vi "Data Readers and Writers.vi"(5 "Calling VI Ref":refnum<vi>, 8 "error in (no error)":errorcluster, 9 "Full Element Name":string[](array[string]), 11 "JKI SM in":refnum<class "JKI SM.lvclass">) -> (0 "error out":errorcluster)   [LabVIEW 2020]
uses:
  <userlib>/_OpenG.lib/comparison/comparison.llb/openg_comparison__ogtk.lvlib
  JKI State Machine API/source/JKI SM/JKI SM.lvclass
  <vilib>/regexp/Match Regular Expression.xnode
  <userlib>/_OpenG.lib/comparison/comparison.llb/I32 Changed__ogtk.vi
  <userlib>/_OpenG.lib/comparison/comparison.llb/Boolean Changed__ogtk.vi
  <userlib>/_OpenG.lib/error/error.llb/openg_error.lvlib
  <userlib>/_OpenG.lib/error/error.llb/Filter Error Codes (Array)__ogtk.vi
  <userlib>/_OpenG.lib/string/string.llb/openg_string.lvlib
panel:
  in  "Listbox":i32(listbox)
  in  "OK":bool
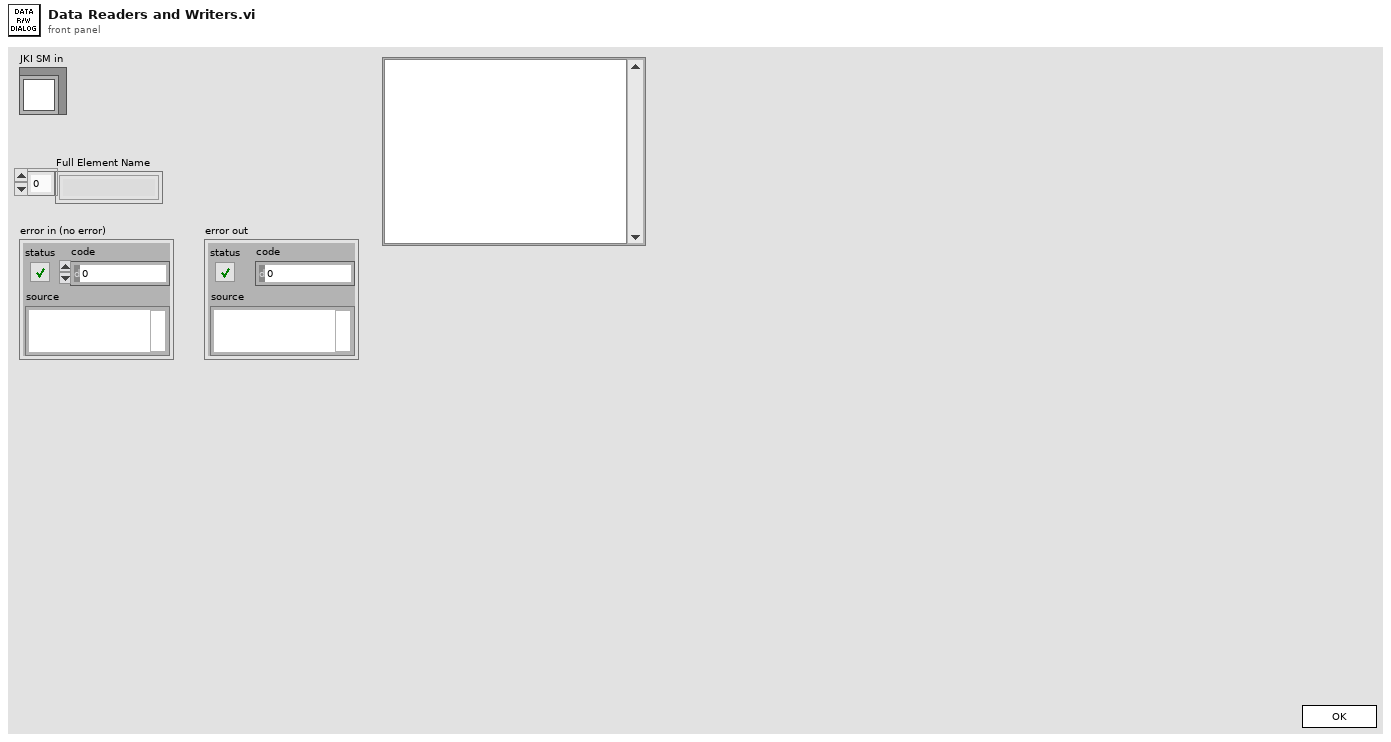
[diagram p1: front panel]
types:
  T1 = enum32{"Invalid", "Standard", "Closed", "Hidden", "Minimized", "Maximized"}
  T2 = enum32{"invalid app kind", "Development System", "Run Time System", "Student Edition", "Embedded LabVIEW", "Evaluation", "Custom"}
  T3 = enum32{"Invalid", "Default", "Floating", "Floating/Auto-Hide", "Modal"}
  T4 = cluster{"Core":cluster{"Current VI Reference":refnum<vi>, "Close Panel on Exit?":bool}, "Your Boolean data":bool, "Your string data":string, "JKI SM in":refnum<class "JKI SM.lvclass">, "Full Element Name":string[]}
  T5 = typedef "LVPoint32TypeDef.ctl" = cluster{"Horizontal":i32, "Vertical":i32}
  T6 = cluster{"Shift":bool, "Ctrl":bool, "Alt":bool, "Cmd":bool, "Opt":bool}
  T7 = cluster{"StringConstant":refnum<vi>, "Structure":string, "Frame Name":string, "State Call":string}[]
  T8 = cluster{"Current VI Reference":refnum<vi>, "Close Panel on Exit?":bool}
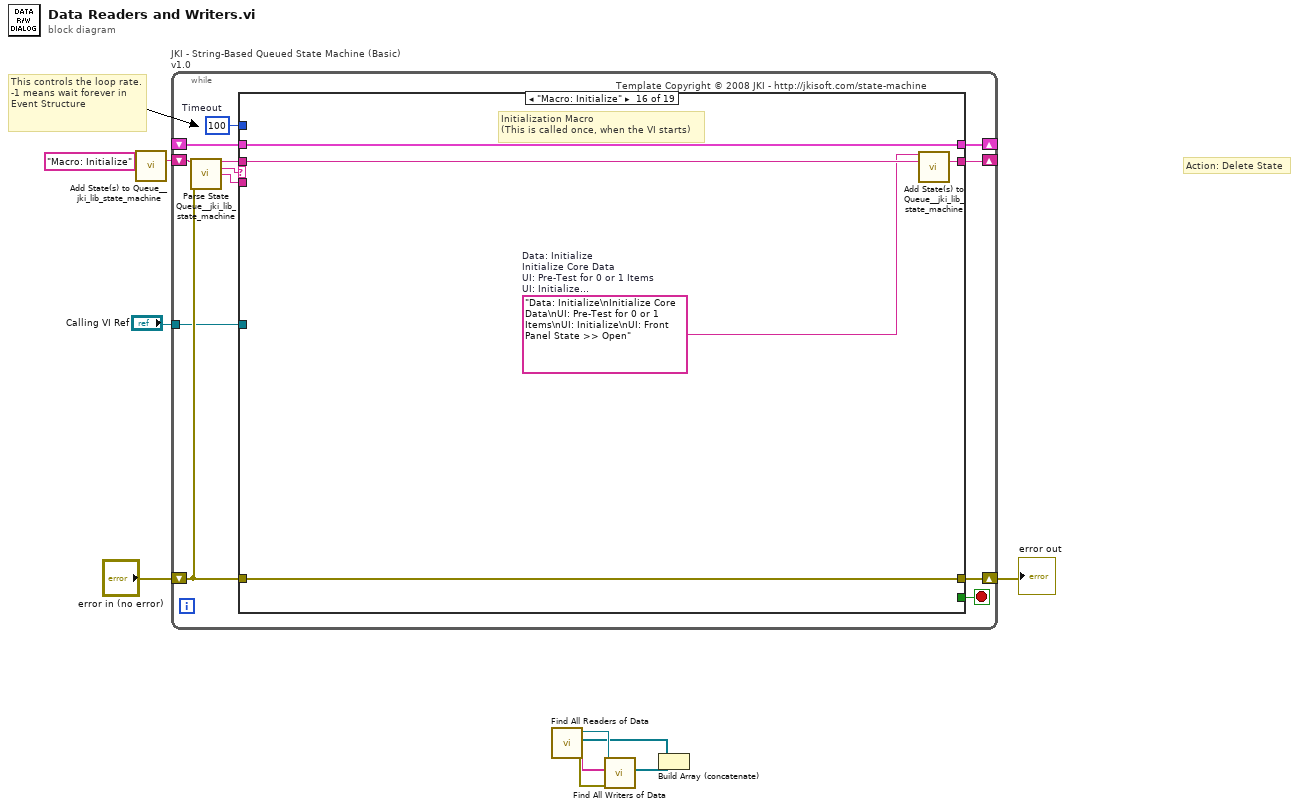
[diagram p0: block diagram]
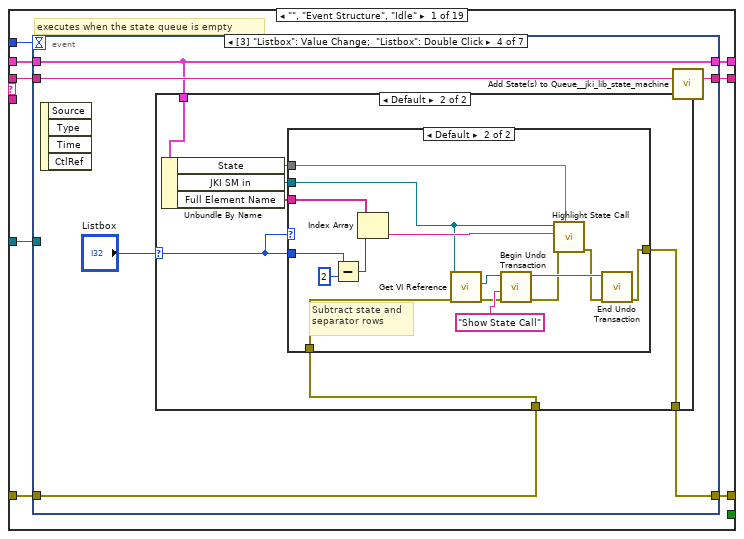
[diagram p2: hidden frame]
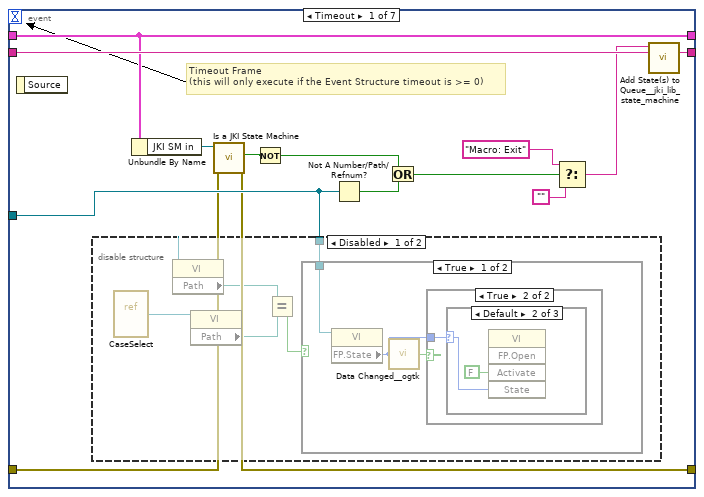
[diagram p3: hidden frame]
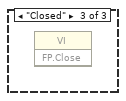
[diagram p6: hidden frame]
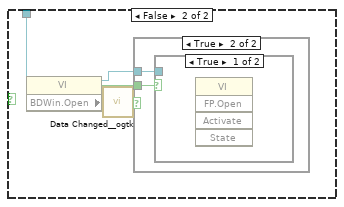
[diagram p7: hidden frame]
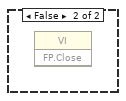
[diagram p9: hidden frame]
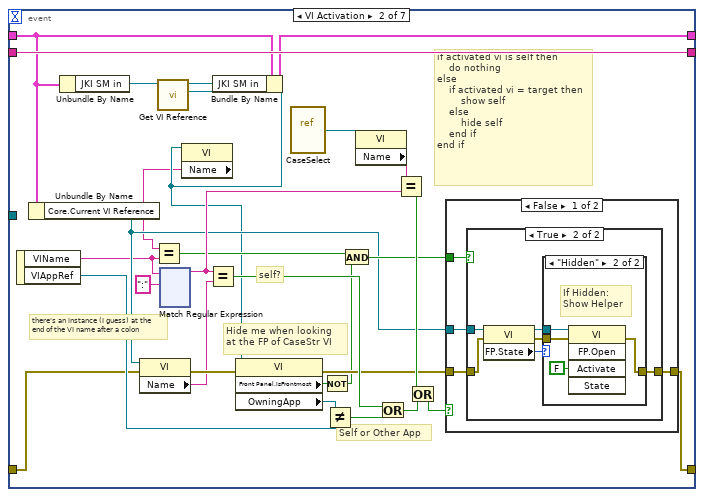
[diagram p11: hidden frame]
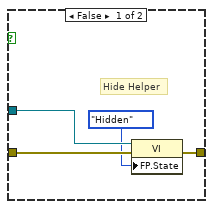
[diagram p12: hidden frame]
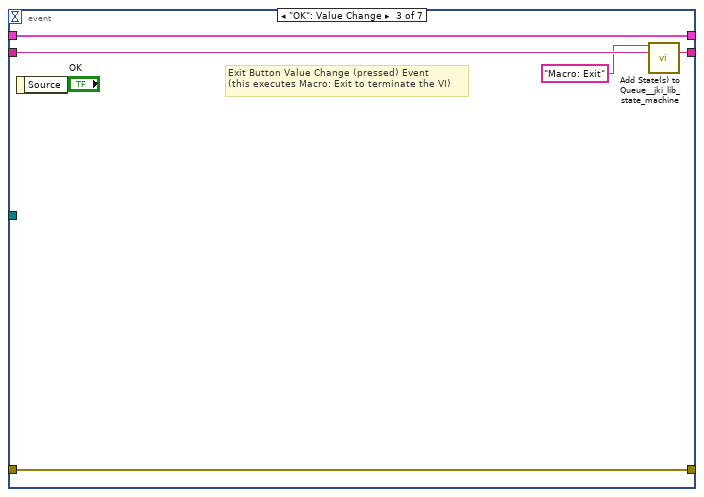
[diagram p15: hidden frame]
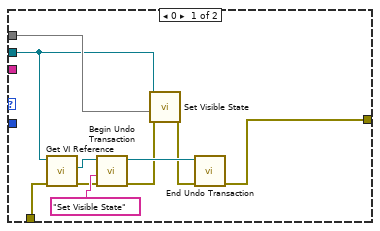
[diagram p17: hidden frame]
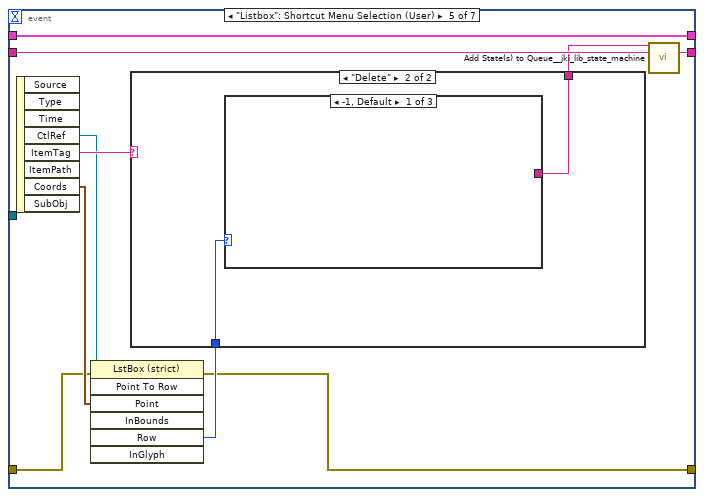
[diagram p18: hidden frame]
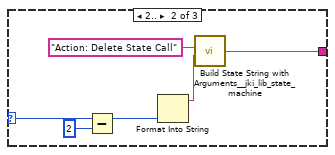
[diagram p20: hidden frame]
diagram:
  # "Action: Delete State"
  # "This controls the loop rate. -1 means wait forever in Event Structure"
  n1 = call <vilib>:"Add State(s) to Queue__jki_lib_state_machine.vi"("State(s) in (\"\")"="Macro: Initialize") -> ("States Out"=w12:string)  [unwired: 14 in]
  n2 = while "JKI - String-Based Queued State Machine (Basic) v1.0" {
    shift-right: [w17] -> _
    shift-left: _ -> [w16]
    shift-right: [w20] -> w10
    shift-left: "error in (no error)" -> [w14]
    shift-right: [w19] -> _
    shift-left: w12 -> [w21]
    tunnel: "Calling VI Ref" -> [w13]
    stop <- w18 stop-if-true
    w15 = 100  # Timeout
    # "Template Copyright © 2008 JKI - http://jkisoft.com/state-machine"
    n3 = call <vilib>:"Parse State Queue__jki_lib_state_machine.vi"("State Queue"=w21, "Error In (no error)"=w14) -> ("Remaining States"=w23:string, "Current State"=w24:string, "Arguments"=w22:string)  [unwired: 11 in]
    n4 = case shown="\"Macro: Initialize\"" w24 {
      selector: w24 -> [_ _ w376 _ _ _ _ _ _ _ _ _ _ _ _ _ _ _ _]
      tunnel: w23 -> [w32 w375 w380 w400 w411 w416 w420 w429 w436 w440 w459 w476 w495 w506 w535 w540 w550 w554 w558]
      tunnel: w22 -> [_ _ _ _ _ _ _ _ _ _ _ _ w490 w500 _ _ _ _ _]
      tunnel: w16 -> [w30 w372 w378 w392 w408 w414 w417 _ w433 w437 w456 w470 w493 w502 w532 w538 w547 w551 w555]
      tunnel: [w29 w373 w382 w387 errorcluster {"status"=FALSE, "code"=0, "source"=""} ("error out") w413 w418 w426 w431 w438 w457 w467 w491 w503 w533 w536 w548 w552 w556] -> w20
      tunnel: w14 -> [w28 w373 w381 w388 w406 w413 w418 w426 w430 w438 w457 w468 w492 w504 w533 w536 w548 w552 w556]
      tunnel: [w31 w374 w379 w399 w410 w415 w419 w428 w435 w439 w458 w475 w494 w505 w534 w539 w549 w553 w557] -> w19
      tunnel: [_ _ _ _ _ TRUE _ _ _ _ _ _ _ _ _ _ _ _ _] -> w18
      tunnel: [w27 w372 w378 w398 w408 w414 w417 w427 w433 w437 w456 w470 w493 w502 w532 w538 w547 w551 w555] -> w17
      tunnel: w15 -> [w26 _ _ _ _ _ _ _ _ _ _ _ _ _ _ _ _ _ _]
      tunnel: w13 -> [w25 _ _ _ _ _ _ _ _ _ _ _ _ _ _ _ _ _ _]
      frame "", "Event Structure", "Idle" {
        # "executes when the state queue is empty"
        n5 = event shown="[3] \"Listbox\": Value Change;  \"Listbox\": Double Click" {
          selector: _ -> [_ _ _ _ _ _ _]
          dyn-events: _ -> [_ _ _ _ _ _ _]
          timeout: w26 -> [_ _ _ _ _ _ _]
          tunnel: w32 -> [w46 w92 w228 w234 w277 w297 w371]
          tunnel: [w45 w92 w227 w233 w276 w296 w370] -> w31
          tunnel: w30 -> [w40 w66 w225 w232 w269 w295 w368]
          tunnel: [w35 w67 w226 w230 w268 w290 w369] -> w29
          tunnel: w28 -> [w36 w68 w226 w231 w271 w291 w369]
          tunnel: [w40 w65 w225 w232 w269 w295 w368] -> w27
          tunnel: w25 -> [w41 _ _ _ _ _ _]
          event Timeout {
            # "Timeout Frame\n(this will only execute if the Event Structure timeout is >= 0)"
            n6 = event-data() -> ()  [unwired: 1 in, 1 out]
            n7 = disable-structure shown="Disabled" {
              disable-tunnel: w41 -> [w47 _]
              frame Disabled {
                n8 = vi-ref "CaseSelect.vi"() -> (w49:refnum<vi>)
                n9 = property class="VI"(reference=w47) -> ("Path"=w48:path)  [unwired: 1 in, 2 out]
                n10 = property class="VI"(reference=w49) -> ("Path"=w51:path)  [unwired: 1 in, 2 out]
                n11 = Equal?(x=w48, y=w51) -> (x = y?=w50:bool)
                n12 = case shown="True" w50 {
                  tunnel: w47 -> [w52 w59]
                  frame True {
                    n13 = property class="VI"(reference=w52) -> ("FP.State"=w53:T1)  [unwired: 1 in, 2 out]
                    n14 = call-poly <userlib>:"Data Changed__ogtk.vi"("I32"=w53) -> ("Changed"=w54:bool)
                    n15 = case shown="True" w54 {
                      tunnel: w53 -> [_ w55]
                      frame False {
                      }
                      frame True {
                        n16 = case shown="Default" w55 {
                          selector: w55 -> [_ w56 _]
                          frame "Invalid" {
                          }
                          frame Default {
                            n17 = invoke class="VI" method="FP.Open"("Activate"=FALSE ("Activate?"), "State"=w56) -> ()  [unwired: 3 in, 5 out]
                          }
                          frame "Closed" {
                            n18 = invoke class="VI" method="FP.Close"() -> ()  [unwired: 3 in, 3 out]
                          }
                        }
                      }
                    }
                  }
                  frame False {
                    n19 = property class="VI"(reference=w59) -> (reference out=w58:refnum<vi>, "BDWin.Open"=w60:bool)  [unwired: 1 in, 1 out]
                    n20 = call-poly <userlib>:"Data Changed__ogtk.vi"("Boolean"=w60) -> ("Changed"=w61:bool)
                    n21 = case shown="True" w61 {
                      tunnel: w60 -> [_ w63]
                      tunnel: w58 -> [_ w62]
                      frame False {
                      }
                      frame True {
                        n22 = case shown="True" w63 {
                          tunnel: w62 -> [_ _]
                          frame True {
                            n23 = invoke class="VI" method="FP.Open"() -> ()  [unwired: 5 in, 5 out]
                          }
                          frame False {
                            n24 = invoke class="VI" method="FP.Close"() -> ()  [unwired: 3 in, 3 out]
                          }
                        }
                      }
                    }
                  }
                }
              }
              frame Enabled {
              }
            }
            n25 = Unbundle By Name(w40) -> ("JKI SM in"=w39:refnum<class "JKI SM.lvclass">)
            n26 = call "Is a JKI State Machine.vi"("error in (no error)"=w36, "JKI SM in"=w39) -> ("error out"=w35:errorcluster, "Is a JKI State Machine"=w38:bool)  [unwired: 7 in, 1 out]
            n27 = Not(x=w38) -> (.not. x?=w37:bool)
            n28 = Not A Number/Path/Refnum?(number/path/refnum=w41) -> (NaN/Path/Refnum?=w34:bool)
            n29 = Or(x=w37, y=w34) -> (x .or. y?=w33:bool)
            n30 = Select(t="Macro: Exit", s=w33, f="") -> (s? t:f=w42:string)
            n31 = call <vilib>:"Add State(s) to Queue__jki_lib_state_machine.vi"("State(s) in Front (\"\")"=w42, "State(s) in (\"\")"=w46) -> ("States Out"=w45:string)  [unwired: 13 in]
          }
          event VI Activation {
            # "Self or Other App"
            # "self?"
            # "Hide me when looking\nat the FP of CaseStr VI"
            # "there's an instance (I guess) at the\nend of the VI name after a colon"
            # "if activated vi is self then\n    do nothing\nelse\n    if activated vi = target then\n        show self\n    else\n        hide self\n    end if\nend if"
            n32 = event-data() -> ("VIName"=w70:string, "VIAppRef"=w69:refnum<vi>)  [unwired: 1 in]
            n33 = Unbundle By Name(w66) -> ("Core.Current VI Reference"=w77:refnum<vi>)
            n34 = Unbundle By Name(w66) -> ("JKI SM in"=w73:refnum<class "JKI SM.lvclass">)
            n35 = property class="VI"(reference=w77, error in=w68) -> (error out=w81:errorcluster, "Name"=w76:string)  [unwired: 1 out]
            n36 = call "Get VI Reference.vi"("JKI SM in"=w73) -> ("VI"=w72:refnum<vi>, "JKI SM out"=w64:refnum<class "JKI SM.lvclass">)  [unwired: 8 in, 1 out]
            n37 = xnode "Match Regular Expression"("input string"=w70, "regular expression"=":") -> ("before match"=w88:string)  [unwired: 3 in, 5 out]
            n38 = property class="VI"(reference=w72) -> ("Name"=w71:string)  [unwired: 1 in, 2 out]
            n39 = Equal?(x=w71, y=w70) -> (x = y?=w74:bool)
            n40 = Equal?(x=w88, y=w76) -> (x = y?=w85:bool)
            n41 = Bundle By Name(cluster=w66, "JKI SM in"=w64) -> (w65:T4)
            n42 = property class="VI"(reference=w72, error in=w81) -> (error out=w80:errorcluster, "Front Panel.IsFrontmost"=w78:bool, "OwningApp"=w83:refnum<vi>)  [unwired: 1 out]
            n43 = vi-ref "CaseSelect.vi"() -> (w86:refnum<vi>)
            n44 = Not(x=w78) -> (.not. x?=w79:bool)
            n45 = Not Equal?(x=w83, y=w69) -> (x != y?=w84:bool)
            n46 = And(x=w74, y=w79) -> (x .and. y?=w82:bool)
            n47 = property class="VI"(reference=w86) -> ("Name"=w87:string)  [unwired: 1 in, 2 out]
            n48 = Or(x=w85, y=w84) -> (x .or. y?=w90:bool)
            n49 = Equal?(x=w87, y=w88) -> (x = y?=w89:bool)
            n50 = Or(x=w89, y=w90) -> (x .or. y?=w91:bool)
            n51 = case shown="False" w91 {
              tunnel: w80 -> [w96 w112]
              tunnel: [w94 w112] -> w67
              tunnel: w77 -> [w95 _]
              tunnel: w82 -> [w93 _]
              frame False {
                n52 = case shown="True" w93 {
                  tunnel: w96 -> [w100 w105]
                  tunnel: w95 -> [w99 w106]
                  tunnel: [w98 w103] -> w94
                  frame False {
                    # "Hide Helper"
                    n53 = property class="VI"(reference=w99, error in=w100, "FP.State"=T1."Hidden" ("Front Panel Window:State")) -> (error out=w98:errorcluster)  [unwired: 1 out]
                  }
                  frame True {
                    n54 = property class="VI"(reference=w106, error in=w105) -> (reference out=w102:refnum<vi>, error out=w101:errorcluster, "FP.State"=w104:T1)
                    n55 = case shown="\"Hidden\"" w104 {
                      tunnel: [w107 w111] -> w103
                      tunnel: w102 -> [_ w110]
                      tunnel: w101 -> [w107 w109]
                      frame Default {
                      }
                      frame "Hidden" {
                        # "If Hidden:\nShow Helper"
                        n56 = invoke class="VI" method="FP.Open"(reference=w110, error in=w109, "Activate"=FALSE ("Activate?")) -> (error out=w111:errorcluster)  [unwired: 2 in, 4 out]
                      }
                    }
                  }
                }
              }
              frame True {
              }
            }
          }
          event "OK": Value Change {
            # "Exit Button Value Change (pressed) Event\n(this executes Macro: Exit to terminate the VI)"
            n57 = event-data() -> ()  [unwired: 1 in, 1 out]
            n58 = call <vilib>:"Add State(s) to Queue__jki_lib_state_machine.vi"("State(s) in Front (\"\")"="Macro: Exit", "State(s) in (\"\")"=w228) -> ("States Out"=w227:string)  [unwired: 13 in]
          }
          event "Listbox": Value Change; "Listbox": Double Click {
            n59 = event-data() -> ()  [unwired: 1 in, 4 out]
            n60 = case shown="Default" "Listbox" {
              selector: "Listbox" -> [_ w236]
              tunnel: w232 -> [_ w242]
              tunnel: w231 -> [w235 w239]
              tunnel: [w235 w238] -> w230
              frame -1 {
              }
              frame Default {
                n61 = Unbundle By Name(w242) -> ("State"=w237, "JKI SM in"=w240:refnum<class "JKI SM.lvclass">, "Full Element Name"=w241:string[])
                n62 = case shown="Default" w236 {
                  tunnel: w241 -> [_ w267]
                  tunnel: w240 -> [w246 w258]
                  tunnel: w239 -> [w247 w254]
                  tunnel: w236 -> [_ w263]
                  tunnel: [w243 w255] -> w238
                  tunnel: w237 -> [w252 w265]
                  frame 0 {
                    n63 = call "Get VI Reference.vi"("error in (no error)"=w247, "JKI SM in"=w246) -> ("error out"=w250:errorcluster, "VI"=w249:refnum<vi>)  [unwired: 7 in, 1 out]
                    n64 = call "Begin Undo Transaction.vi"("error in (no error)"=w250, "Action"="Set Visible State", "VI in"=w249) -> ("error out"=w245:errorcluster, "VI out"=w248:refnum<vi>)  [unwired: 7 in]
                    n65 = call "Set Visible State.vi"("error in (no error)"=w245, "State Name"=w252, "JKI SM in"=w246) -> ("error out"=w244:errorcluster)  [unwired: 7 in, 1 out]
                    n66 = call "End Undo Transaction.vi"("error in (no error)"=w244, "VI in"=w248) -> ("error out"=w243:errorcluster)  [unwired: 8 in, 1 out]
                  }
                  frame Default {
                    # "Subtract state and separator rows"
                    n67 = Subtract(x=w263, y=2) -> (x-y=w262:i32)
                    n68 = Index Array(array=w267, index=w262) -> (element=w266:string)
                    n69 = call "Get VI Reference.vi"("error in (no error)"=w254, "JKI SM in"=w258) -> ("error out"=w260:errorcluster, "VI"=w259:refnum<vi>)  [unwired: 7 in, 1 out]
                    n70 = call "Begin Undo Transaction.vi"("error in (no error)"=w260, "Action"="Show State Call", "VI in"=w259) -> ("error out"=w253:errorcluster, "VI out"=w257:refnum<vi>)  [unwired: 7 in]
                    n71 = call "Highlight State Call.vi"(7:w265, "error in (no error)"=w253, "State Call"=w266, "JKI SM in"=w258) -> ("error out"=w256:errorcluster)  [unwired: 6 in, 1 out]
                    n72 = call "End Undo Transaction.vi"("error in (no error)"=w256, "VI in"=w257) -> ("error out"=w255:errorcluster)  [unwired: 8 in, 1 out]
                  }
                }
              }
            }
            n73 = call <vilib>:"Add State(s) to Queue__jki_lib_state_machine.vi"("State(s) in (\"\")"=w234) -> ("States Out"=w233:string)  [unwired: 14 in]
          }
          event "Listbox": Shortcut Menu Selection (User) {
            n74 = event-data() -> ("CtlRef"=w274:refnum<vi>, "ItemTag"=w275:string, "Coords"=w273:T5)  [unwired: 1 in, 5 out]
            n75 = invoke class="LstBox (strict)" method="Point To Row"(reference=w274, error in=w271, "Point"=w273) -> (error out=w268:errorcluster, "Row"=w272:i32)  [unwired: 4 in, 5 out]
            n76 = case shown="\"Delete\"" w275 {
              tunnel: w272 -> [_ w279]
              tunnel: [_ w278] -> w270
              frame Default {
              }
              frame "Delete" {
                n77 = case shown="-1, Default" w279 {
                  selector: w279 -> [_ w282 _]
                  tunnel: [_ w283 w286] -> w278
                  frame -1, Default {
                  }
                  frame 2.. {
                    n78 = Subtract(x=w282, y=2) -> (x-y=w281:i32)
                    n79 = Format Into String(w281) -> (resulting string=w284:string)  [unwired: 3 in, 1 out]
                    n80 = call <vilib>:"Build State String with Arguments__jki_lib_state_machine.vi"("Arguments (\"\")"=w284, "State"="Action: Delete State Call") -> ("State with Arguments"=w283:string)  [unwired: 4 in]
                  }
                  frame 0 {
                    n81 = call <vilib>:"Build State String with Arguments__jki_lib_state_machine.vi"("State"="Action: Delete State") -> ("State with Arguments"=w286:string)  [unwired: 5 in]
                  }
                }
              }
            }
            n82 = call <vilib>:"Add State(s) to Queue__jki_lib_state_machine.vi"("State(s) in Front (\"\")"=w270, "State(s) in (\"\")"=w277) -> ("States Out"=w276:string)  [unwired: 13 in]
          }
          event Key Down? {
            n83 = event-data() -> ("Char"=w294:i16, "ScanCode"=w289:i16, "PlatMods"=w293:T6)  [unwired: 1 in, 7 out]
            n84 = case shown="Default" w289 {
              tunnel: w295 -> [_ w315]
              tunnel: w294 -> [_ w313]
              tunnel: w293 -> [_ w310]
              tunnel: [_ w308] -> w292
              tunnel: w291 -> [w299 w306]
              tunnel: [w299 w305] -> w290
              tunnel: [w298 _] -> w288
              frame 83 {
                n85 = local read "Listbox"() -> (w300:i32)
                n86 = case shown="Default" w300 {
                  selector: w300 -> [_ w301]
                  tunnel: [_ w302] -> w298
                  frame -1 {
                  }
                  frame Default {
                    n87 = Format Into String(w301) -> (resulting string=w303:string)  [unwired: 3 in, 1 out]
                    n88 = call <vilib>:"Build State String with Arguments__jki_lib_state_machine.vi"("Arguments (\"\")"=w303, "State"="Action: Delete State Call") -> ("State with Arguments"=w302:string)  [unwired: 4 in]
                  }
                }
              }
              frame Default {
                n89 = Unbundle By Name(w315) -> ("JKI SM in"=w307:refnum<class "JKI SM.lvclass">, "Full Element Name"=w314:string[])
                n90 = Build Array(w313) -> (w312:i16[])
                n91 = Unbundle By Name(w310) -> ("Ctrl"=w309:bool)
                n92 = Byte Array To String(unsigned byte array=w312) -> (string=w311:string)
                n93 = case shown="True" w309 {
                  tunnel: w314 -> [_ w324]
                  tunnel: w311 -> [_ w323]
                  tunnel: w310 -> [_ w322]
                  tunnel: [_ w321] -> w308
                  tunnel: w307 -> [_ w319]
                  tunnel: [w316 w318] -> w305
                  tunnel: w306 -> [w316 w317]
                  frame False {
                  }
                  frame True {
                    n94 = To Upper Case(1:w323) -> (0:w320:string)
                    n95 = case shown="\"Z\"" w320 {
                      tunnel: w324 -> [_ w339 w349 _]
                      tunnel: w322 -> [_ w334 _ w358]
                      tunnel: [_ TRUE TRUE TRUE] -> w321
                      tunnel: w319 -> [_ _ w342 w355]
                      tunnel: [w325 w332 w340 w352] -> w318
                      tunnel: w317 -> [w325 w332 w341 w356]
                      frame Default {
                      }
                      frame "G" {
                        w327 = 2 ("y")
                        n96 = local read "Listbox"() -> (w329:i32)
                        n97 = Unbundle By Name(w334) -> ("Shift"=w335:bool)
                        n98 = Array Size(array=w339) -> (size(s)=w326:i32)
                        n99 = Subtract(x=w329, y=w327) -> (x-y=w328:i32)
                        n100 = Decrement(x=w328) -> (x-1=w337:i32)
                        n101 = Increment(x=w328) -> (x+1=w338:i32)
                        n102 = Select(t=w337, s=w335, f=w338) -> (s? t:f=w336:i32)
                        n103 = Quotient & Remainder(x=w336, y=w326) -> (x-y*floor(x/y)=w331:i32)  [unwired: 1 out]
                        n104 = Add(x=w331, y=w327) -> (x+y=w330:i32)
                        n105 = property on="Listbox" class="LstBox (strict)"("Val(Sgnl)"=w330) -> ()  [unwired: 2 in, 2 out]
                      }
                      frame "F" {
                        n106 = local read "Listbox"() -> (w350:i32)
                        n107 = Index Array(array=w349, index=w350) -> (element=w348:string)
                        n108 = Unbundle By Name(w348) -> ("Frame Name"=w344)
                        n109 = control-ref of="This VI"() -> (w343:refnum<vi>)
                        n110 = call "Find All Callers of State.vi"("error in (no error)"=w341, "State Name"=w344, "JKI SM in"=w342) -> ("error out"=w345:errorcluster, "Callers"=w346:T7, "JKI SM out"=w347:refnum<class "JKI SM.lvclass">)  [unwired: 6 in]
                        n111 = call "Open Search Results Dialog.vi"("VI Refnum"=w343, "error in (no error)"=w345, "Callers"=w346, "State"=w344, "JKI SM in"=w347) -> ("error out"=w340:errorcluster)  [unwired: 6 in]
                      }
                      frame "Z" {
                        # "Override Ctrl+Z and Ctrl+Shift+Z\n(Handle them here and target the user's VI)"
                        n112 = call "Get VI Reference.vi"("error in (no error)"=w356, "JKI SM in"=w355) -> ("error out"=w353:errorcluster, "VI"=w354:refnum<vi>)  [unwired: 7 in, 1 out]
                        n113 = Unbundle By Name(w358) -> ("Shift"=w357:bool)
                        n114 = case shown="False" w357 {
                          tunnel: w354 -> [w362 w365]
                          tunnel: w353 -> [w360 w364]
                          tunnel: [w361 w363] -> w352
                          frame False {
                            n115 = invoke class="VI" method="Transaction.Undo"(reference=w362, error in=w360) -> (error out=w361:errorcluster)  [unwired: 1 in, 2 out]
                          }
                          frame True {
                            n116 = invoke class="VI" method="Transaction.Redo"(reference=w365, error in=w364) -> (error out=w363:errorcluster)  [unwired: 1 in, 2 out]
                          }
                        }
                      }
                    }
                  }
                }
              }
            }
            n117 = event-data("Discard?"=w292) -> ()  [unwired: 1 in, 1 out]
            n118 = call <vilib>:"Add State(s) to Queue__jki_lib_state_machine.vi"("State(s) in Front (\"\")"=w288, "State(s) in (\"\")"=w297) -> ("States Out"=w296:string)  [unwired: 13 in]
          }
          event Panel Close? {
            # "Discard the event because we'll close the front panel ourselves in Macro: Exit"
            # "Close Panel button (pressed) Event\n(this executes Macro: Exit to terminate the VI)"
            n119 = event-data() -> ()  [unwired: 1 in, 1 out]
            n120 = event-data("Discard?"=TRUE) -> ()  [unwired: 1 in, 1 out]
            n121 = call <vilib>:"Add State(s) to Queue__jki_lib_state_machine.vi"("State(s) in Front (\"\")"="Macro: Exit", "State(s) in (\"\")"=w371) -> ("States Out"=w370:string)  [unwired: 13 in]
          }
        }
      }
      frame "---------- Core ----------" {
        # "Do not put any code in this frame.\n(it is a separator no-op)"
        n122 = call <vilib>:"Add State(s) to Queue__jki_lib_state_machine.vi"("State(s) in (\"\")"=w375) -> ("States Out"=w374:string)  [unwired: 14 in]
      }
      frame Default {
        w385 = 42 items=["No error", "Argument error", "Memory is full", "Out of zone", "End of file", "File already open", "Generic file I/O error", "File not found", "File permission error", "Disk is full", "Duplicate path", "Too many files open", "System feature not enabled", "Resource file not found", "Cannot add resource", "Resource not found", "Image not found", "Image memory error", "Pen does not exist", "Config type invalid", "Config token not found", "Config parse error", "Config memory error", "Bad external code format", "Bad external code offset", "External code not present", "Null window", "Destroy window error", "Null menu", "Print aborted", "Bad print record", "Print driver error", "Windows error during printing", "Memory error during printing", "Print dialog error", "Generic print error", "Invalid device refnum", "Device not found", "Device parameter error", "Device unit error", "Cannot open device", "Device call aborted", "Generic error", "Cancelled by user", "Object ID too low", "Object ID too high", "Object not in heap", "Unknown heap", "Unknown object (invalid DefProc)", "Unknown object (DefProc not in table)", "Message out of range", "Invalid (null) method", "Unknown message", "Manager call not supported", "Bad address", "Network operation in progress", "Network operation timed out", "Connection is busy", "Network attribute not supported", "Network error", "Address in use", "System out of memory", "Connection aborted", "Connection refused", "Not connected", "Already connected", "Connection closed", "Initialization error (interapplication manager)", "Bad occurrence", "Wait on unbound occurrence handler", "Occurrence queue overflow", "Datalog type conflict", "Unused", "Unrecognized type (interapplication manager)", "Memory corrupt", "Failed to make temporary DLL", "Old CIN version", "Drag socket not found", "Failed to load drop-object", "Failed to register OLE object", "Failed to release OLE object", "Format specifier type mismatch", "Unknown format specifier", "Too few format specifiers", "Too many format specifiers", "Scan failed", "Newer CIN version", "Error converting to variant", "Runtime menu error", "Password tampered", "Variant attribute not found", "Incompatible variant data type", "Event data is not available", "Event Store is not present", "Occurrence is not found", "Event Queue is not created", "Event info is not available", "Refnum passed is NULL", "Error retrieving Class GUID", "Error retrieving CoClass GUID", "Error retrieving TypeLib GUID.", "Bad built application magic bytes.", "Specific driver is different from the specific driver associated with the Logical Name.", "There is no session opened to the class driver.", "Max Error", "MAX - Error with config objects", "MAX - Error loading configuration", "MAX - Group not supported"]
        # "Current State"
        # "Do not delete, rename, or modify this frame.\n(this is used to capture unhandled states and typos)"
        # "Handle mistyped state name (developer tool)"
        n123 = Format Into String(format string="Software Exception: Unhandled State \"%s\"." ("message"), error in=w381, w376) -> (resulting string=w384:string, error out=w383:errorcluster)  [unwired: 1 in]
        n124 = call <vilib>:"Error Cluster From Error Code.vi"("show call chain? (False)"=TRUE, "error in (no error)"=w383, "error message (\"\")"=w384, "error code (0)"=w385) -> ("error out"=w382:errorcluster)  [unwired: 5 in]
        n125 = call <vilib>:"Add State(s) to Queue__jki_lib_state_machine.vi"("State(s) in (\"\")"=w380) -> ("States Out"=w379:string)  [unwired: 14 in]
      }
      frame "Initialize Core Data" {
        # "Do not delete, rename, or modify this frame.\n(this is used to determine panel behavior on exit)"
        # "originally closed?"
        # "exe?"
        # "If panel starts closed or is an EXE, then close it when we exit"
        n126 = property class="VI"() -> ("Clone Name"=w390:string)  [unwired: 2 in, 2 out]
        n127 = Open VI Reference(vi path=w390, error in (no error)=w388) -> (vi reference=w389:refnum<vi>, error out=w387:errorcluster)  [unwired: 4 in]
        n128 = property class="VI"() -> ("Front Panel.Open"=w397:bool)  [unwired: 2 in, 2 out]
        n129 = property class="App"() -> ("App.Kind"=w396:T2)  [unwired: 2 in, 2 out]
        n130 = Not(x=w397) -> (.not. x?=w394:bool)
        n131 = Equal?(x=w396, y=T2."Run Time System" ("Application:Kind")) -> (x = y?=w393:bool)
        n132 = Or(x=w394, y=w393) -> (x .or. y?=w391:bool)
        n133 = Bundle By Name(cluster=w392, "Core.Current VI Reference"=w389, "Core.Close Panel on Exit?"=w391) -> (w398:T4)
        n134 = call <vilib>:"Add State(s) to Queue__jki_lib_state_machine.vi"("State(s) in (\"\")"=w400) -> ("States Out"=w399:string)  [unwired: 14 in]
      }
      frame "Error Handler" {
        w407 = i32[] [1026]  # JKI SM VI Invalid Ref
        # "Unhandled Error -- Display it"
        # "Handle any errors here.\nYou can also output any states to clean-up after errors occur"
        # "Clear error"
        n135 = call-poly <userlib>:"Filter Error Codes__ogtk.vi"("Error In"=w406, "Error Codes to Filter"=w407) -> ("Error Out"=w405:errorcluster, "Error Filtered?"=w404:bool)  [unwired: 7 in, 1 out]
        n136 = call <vilib>:"General Error Handler.vi"("error in (no error)"=w405) -> ()  [unwired: 10 in, 5 out]
        n137 = Select(t="Macro: Exit", s=w404, f="") -> (s? t:f=w401:string)
        n138 = call <vilib>:"Add State(s) to Queue__jki_lib_state_machine.vi"("State(s) in Front (\"\")"=w401, "State(s) in (\"\")"=w411) -> ("States Out"=w410:string)  [unwired: 13 in]
      }
      frame "Exit" {
        # "Do not put any code in this frame.\n(No errors that occur here will be handled.)"
        n139 = call <vilib>:"Add State(s) to Queue__jki_lib_state_machine.vi"("State(s) in (\"\")"=w416) -> ("States Out"=w415:string)  [unwired: 14 in]
      }
      frame "---------- Data ----------" {
        # "Do not put any code in this frame.\n(It is a separator no-op. You can make a copy of this frame to create a new Data frame)"
        n140 = call <vilib>:"Add State(s) to Queue__jki_lib_state_machine.vi"("State(s) in (\"\")"=w420) -> ("States Out"=w419:string)  [unwired: 14 in]
      }
      frame "Data: Initialize" {
        w423 = T8 {"Current VI Reference"=refnum, "Close Panel on Exit?"=FALSE}  # Core
        w425 = TRUE  # Your Boolean data
        w424 = ""  # Your string data
        # "do not delete - used by framework"
        # "Expand Bundle to add new data elements to shift register data."
        # "Add new data here."
        # "Data names and types of shift register data are defined by this bundle."
        # "Initialize the shift-register data, here.\n(data names are defined by what you wire into the bundle function)"
        n141 = Bundle("Core"=w423, "Your Boolean data"=w425, "Your string data"=w424, "JKI SM in"="JKI SM in", "Full Element Name"="Full Element Name") -> (w427:T4)  [unwired: 1 in]
        n142 = call <vilib>:"Add State(s) to Queue__jki_lib_state_machine.vi"("State(s) in (\"\")"=w429) -> ("States Out"=w428:string)  [unwired: 14 in]
      }
      frame "Data: Cleanup" {
        # "Ignore Errors\n(e.g. reference already invalid)"
        # "Cleanup any data and references, here.\n(this is called automatically, by the Macro: Exit)"
        n143 = Unbundle By Name(w433) -> ("Core.Current VI Reference"=w434:refnum<vi>)
        n144 = Close Reference(reference=w434, error in (no error)=w430) -> (error out=w432:errorcluster)
        n145 = Merge Errors(w432, w430) -> (w431:errorcluster)
        n146 = call <vilib>:"Add State(s) to Queue__jki_lib_state_machine.vi"("State(s) in (\"\")"=w436) -> ("States Out"=w435:string)  [unwired: 14 in]
      }
      frame "---------- UI ----------" {
        # "Do not put any code in this frame.\n(It is a separator no-op. You can make a copy of this frame to create a new UI frame)"
        n147 = call <vilib>:"Add State(s) to Queue__jki_lib_state_machine.vi"("State(s) in (\"\")"=w440) -> ("States Out"=w439:string)  [unwired: 14 in]
      }
      frame "UI: Initialize" {
        # "Initialize the User Interface, here.\n(this is called automatically, by the Macro: Init)"
        n148 = Unbundle By Name(w456) -> ("Core.Current VI Reference"=w455:refnum<vi>, "Full Element Name"=w443:string[])
        n149 = call <userlib>:"1D Array to String__ogtk.vi"("delimiter (Tab)"="::", "Array of Strings"=w443) -> ("delimited string"=w441:string)  [unwired: 9 in]
        n150 = disable-structure shown="Disabled" {
          disable-tunnel: [w461 _] -> w449
          disable-tunnel: w443 -> [w460 _]
          frame Disabled {
            n151 = for {
              tunnel: w460 -> [w466] mode=indexing
              tunnel: [w463] -> w461 mode=indexing
              n152 = Unbundle By Name(w466) -> ("Structure"=w465, "Frame Name"=w464)
              n153 = Format Into String(format string="%s: %s", w465, w464) -> (resulting string=w463:string)  [unwired: 2 in, 1 out]
            }
          }
          frame Enabled {
          }
        }
        n154 = Format Into String(format string="Accessors of \"%s\"", w441) -> (resulting string=w453:string)  [unwired: 2 in, 1 out]
        n155 = property class="VI"(reference=w455, "Front Panel.Title"=w453) -> ()  [unwired: 1 in, 2 out]
        n156 = Build Array (concatenate)(w441, "" ("format string"), w449) -> (w450:string[])
        n157 = property on="Listbox" class="LstBox (strict)"("Item Names"=w450, "Value"=-1 ("Listbox")) -> (error out=w448:errorcluster, "Item Symbols"=w447:i32[])  [unwired: 2 in, 1 out]
        n158 = Replace Array Subset(array=w447, new element=-1 ("new element/subarray"), index=1) -> (w446:i32[])
        n159 = property on="Listbox" class="LstBox (strict)"(error in=w448, "Item Symbols"=w446) -> ()  [unwired: 1 in, 2 out]
        n160 = call <vilib>:"Add State(s) to Queue__jki_lib_state_machine.vi"("State(s) in (\"\")"=w459) -> ("States Out"=w458:string)  [unwired: 14 in]
      }
      frame "UI: Pre-Test for 0 or 1 Items" {
        n161 = Unbundle By Name(w470) -> ("JKI SM in"=w471:refnum<class "JKI SM.lvclass">, "State"=w473, "Full Element Name"=w472:string[])
        n162 = Array Size(array=w472) -> (size(s)=w474:i32)
        n163 = case shown="1" w474 {
          tunnel: w473 -> [_ w482 w483]
          tunnel: [_ "Macro: Exit" "Macro: Exit"] -> w469
          tunnel: w472 -> [_ _ w488]
          tunnel: w471 -> [_ _ w487]
          tunnel: w468 -> [w477 w478 w485]
          tunnel: [w477 w478 w484] -> w467
          frame Default {
          }
          frame 0 {
            n164 = Format Into String(format string="State %s has no callers.", w482) -> (resulting string=w480:string)  [unwired: 2 in, 1 out]
            n165 = One Button Dialog(message=w480) -> ()  [unwired: 1 in, 1 out]
          }
          frame 1 {
            n166 = Index Array(array=w488) -> (element=w486:string)  [unwired: 1 in]
            n167 = call "Highlight State Call.vi"(7:w483, "error in (no error)"=w485, "State Call"=w486, "JKI SM in"=w487) -> ("error out"=w484:errorcluster)  [unwired: 6 in, 1 out]
          }
        }
        n168 = call <vilib>:"Add State(s) to Queue__jki_lib_state_machine.vi"("State(s) in Front (\"\")"=w469, "State(s) in (\"\")"=w476) -> ("States Out"=w475:string)  [unwired: 13 in]
      }
      frame "UI: Cursor Set" {
        # "Argument"
        # "Set and Unset Cursor Busy.\n(Usage: \"UI: Cursor Set >> Busy|Idle\")"
        n169 = case shown="\"Idle\", Default" w490 {
          tunnel: w492 -> [w497 w499]
          tunnel: [w496 w498] -> w491
          frame "Idle", Default {
            n170 = call <vilib>:"Unset Busy.vi"("error in (no error)"=w497) -> ("error out"=w496:errorcluster)  [unwired: 10 in]
          }
          frame "Busy" {
            n171 = call <vilib>:"Set Busy.vi"("error in (no error)"=w499) -> ("error out"=w498:errorcluster)  [unwired: 9 in, 1 out]
          }
        }
        n172 = call <vilib>:"Add State(s) to Queue__jki_lib_state_machine.vi"("State(s) in (\"\")"=w495) -> ("States Out"=w494:string)  [unwired: 14 in]
      }
      frame "UI: Front Panel State" {
        # "Argument"
        # "Set Front Panel Open or Closed\n(Usage: \"UI: Front Panel State >> Open|Close\")"
        n173 = Unbundle By Name(w502) -> ("Core.Current VI Reference"=w501:refnum<vi>)
        n174 = case shown="\"Open\", Default" w500 {
          tunnel: w504 -> [w510 w526]
          tunnel: [w512 w527] -> w503
          tunnel: w501 -> [w511 w524]
          frame "Open", Default {
            n175 = property class="VI"(reference=w511, error in=w510) -> (reference out=w508:refnum<vi>, error out=w509:errorcluster, "Front Panel.Open"=w507:bool)
            n176 = case shown="False" w507 {
              tunnel: [w515 w521] -> w512
              tunnel: w509 -> [w518 w521]
              tunnel: w508 -> [w517 _]
              frame False {
                # "Setting Floatin here, instead of VI Properties allows the VI to accept keyboard input immediately after openning. (setting it in VI Properties was causing a bug where it wouldn't receive keyboard input until clicking on the VI)"
                n177 = invoke class="VI" method="FP.Open"(reference=w517, error in=w518, "Activate"=TRUE, "State"=T1."Standard") -> (reference out=w514:refnum<vi>, error out=w516:errorcluster)  [unwired: 1 in, 3 out]
                n178 = property class="VI"(reference=w514, error in=w516, "FP.Behavior"=T3."Floating" ("Front Panel Window:Behavior")) -> (error out=w515:errorcluster)  [unwired: 1 out]
              }
              frame True {
              }
            }
          }
          frame "Close" {
            n179 = property class="VI"(reference=w524, error in=w526) -> (reference out=w523:refnum<vi>, error out=w525:errorcluster, "Front Panel.Open"=w522:bool)
            n180 = case shown="True" w522 {
              tunnel: [w528 w531] -> w527
              tunnel: w525 -> [w528 w530]
              tunnel: w523 -> [_ w529]
              frame False {
              }
              frame True {
                n181 = invoke class="VI" method="FP.Close"(reference=w529, error in=w530) -> (error out=w531:errorcluster)  [unwired: 1 in, 2 out]
              }
            }
          }
        }
        n182 = call <vilib>:"Add State(s) to Queue__jki_lib_state_machine.vi"("State(s) in (\"\")"=w506) -> ("States Out"=w505:string)  [unwired: 14 in]
      }
      frame "---------- Macro ----------" {
        # "Do not put any code in this frame.\n(It is a separator no-op. You can make a copy of this frame to create a new Macro frame)"
        n183 = call <vilib>:"Add State(s) to Queue__jki_lib_state_machine.vi"("State(s) in (\"\")"=w535) -> ("States Out"=w534:string)  [unwired: 14 in]
      }
      frame "Macro: Initialize" {
        w537 = "Data: Initialize\nInitialize Core Data\nUI: Pre-Test for 0 or 1 Items\nUI: Initialize\nUI: Front Panel State >> Open"  # Data: Initialize Initialize Core Data UI: Pre-Test for 0 or 1 Items UI: Initialize UI: Front Panel State >> Open
        # "Initialization Macro\n(This is called once, when the VI starts)"
        n184 = call <vilib>:"Add State(s) to Queue__jki_lib_state_machine.vi"("State(s) in Front (\"\")"=w537, "State(s) in (\"\")"=w540) -> ("States Out"=w539:string)  [unwired: 13 in]
      }
      frame "Macro: Exit" {
        # "Exit Macro\n(This is called once, when the VI exits)"
        n185 = Unbundle By Name(w547) -> ("Core.Close Panel on Exit?"=w546:bool)
        n186 = Select(t="UI: Front Panel State >> Close", s=w546, f="") -> (s? t:f=w543:string)
        n187 = call <vilib>:"Add State(s) to Queue__jki_lib_state_machine.vi"("State(s) in (\"\")"=w543, "State(s) at Back (\"\")"="Data: Cleanup\nExit") -> ("States Out"=w541:string)  [unwired: 13 in]
        n188 = call <vilib>:"Add State(s) to Queue__jki_lib_state_machine.vi"("State(s) in Front (\"\")"=w541, "State(s) in (\"\")"=w550) -> ("States Out"=w549:string)  [unwired: 13 in]
      }
      frame "---------- Action ----------" {
        # "Template Separator\n(You can make a copy of, or modify, this frame)"
        n189 = call <vilib>:"Add State(s) to Queue__jki_lib_state_machine.vi"("State(s) in (\"\")"=w554) -> ("States Out"=w553:string)  [unwired: 14 in]
      }
      frame "New Category: 2" {
        # "Your code here.\n(You can make a copy of, or modify, this frame)"
        n190 = call <vilib>:"Add State(s) to Queue__jki_lib_state_machine.vi"("State(s) in (\"\")"=w558) -> ("States Out"=w557:string)  [unwired: 14 in]
      }
    }
  }
  "error out" <- w10
  n191 = call "Find All Readers of Data.vi"() -> ("error out"=w6:errorcluster, "NamedUnbundlers"=w4:refnum<vi>[], "JKI SM out"=w7:refnum<class "JKI SM.lvclass">, "Full Element Name"=w3:string[])  [unwired: 8 in]
  n192 = call "Find All Writers of Data.vi"("error in (no error)"=w6, "Full Element Name"=w3, "JKI SM in"=w7) -> ("error out"=w1:errorcluster, "NamedBundlers"=w5:refnum<vi>[], "JKI SM out"=w2:refnum<class "JKI SM.lvclass">)  [unwired: 5 in, 1 out]
  n193 = Build Array (concatenate)(w4, w5) -> ()  [unwired: 1 out]
